vi "Create DC Waveforms.vi"(6 "sampling":T1, 8 "error in (no error)":errorcluster, 11 "DC (V)":dbl[](array[numeric])) -> (0 "Error out":errorcluster, 3 "Waveforms []":waveform(dbl)[](array[waveform]))   [LabVIEW 2019, in "Lockin.DAQ.lvclass"]
uses:
  Lockin.DAQ.lvclass
  Typedefs/Sampling.ctl
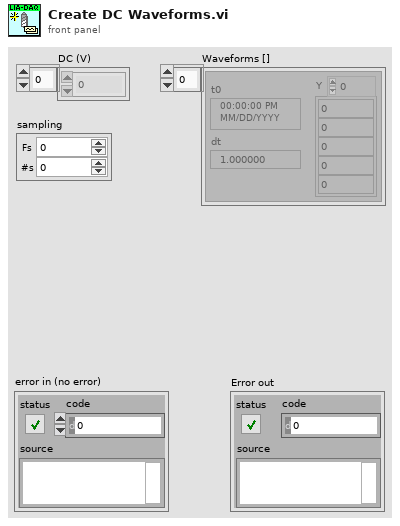
[diagram p1: front panel]
types:
  T1 = typedef "Lockin.DAQ.lvclass/Sampling.ctl" = cluster{"Fs":dbl, "#s":i32}
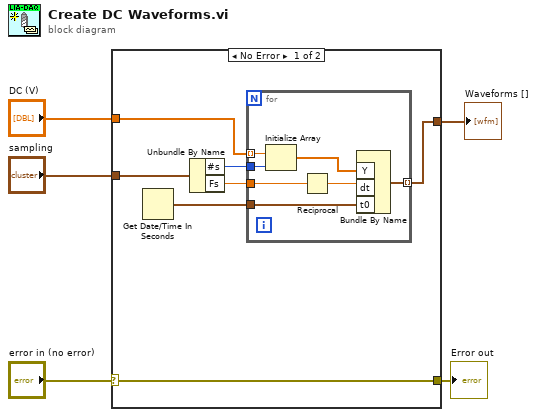
[diagram p0: block diagram]
diagram:
  n1 = case shown="No Error" "error in (no error)" {
    selector: "error in (no error)" -> [w6 w20]
    tunnel: [w12 _] -> w5
    tunnel: "sampling" -> [w11 _]
    tunnel: "DC (V)" -> [w10 _]
    tunnel: [w6 w20] -> w1
    frame No Error {
      n2 = Get Date/Time In Seconds() -> (seconds since 1Jan1904=w9:timestamp)
      n3 = Unbundle By Name(w11) -> ("#s"=w7:i32, "Fs"=w8:dbl)
      n4 = for {
        tunnel: w7 -> [w18]
        tunnel: w10 -> [w19] mode=indexing
        tunnel: w8 -> [w16]
        tunnel: w9 -> [w14]
        tunnel: [w13] -> w12 mode=indexing
        n5 = Initialize Array(w19, w18) -> (w15:dbl[])
        n6 = Reciprocal(x=w16) -> (1/x=w17:dbl)
        n7 = Bundle By Name("Y"=w15, "dt"=w17, "t0"=w14) -> (w13:waveform(dbl))  [unwired: 1 in]
      }
    }
    frame Error {
    }
  }
  "Waveforms []" <- w5
  "Error out" <- w1
